vi "Monitor Torque 2.vi"(0 "reference in":refnum<class "SmartMotor.lvclass">, 3 "Monitoring Duration (ms)":u32, 4 "Torque Limit":i32, 5 "error in (no error)":errorcluster) -> (14 "reference out":refnum<class "SmartMotor.lvclass">, 18 "Limit Passed":bool, 19 "error out":errorcluster)   [LabVIEW 2017, in "SmartMotor.lvclass"]
uses:
  SmartMotor.lvclass
  <vilib>/Analysis/baseanly.llb/Mean (DBL).vi
  <vilib>/Analysis/NI_AALBase.lvlib
panel:
  out "Absolute Motor Torque":dbl(graph)
  out "Max Absolute Torque":dbl
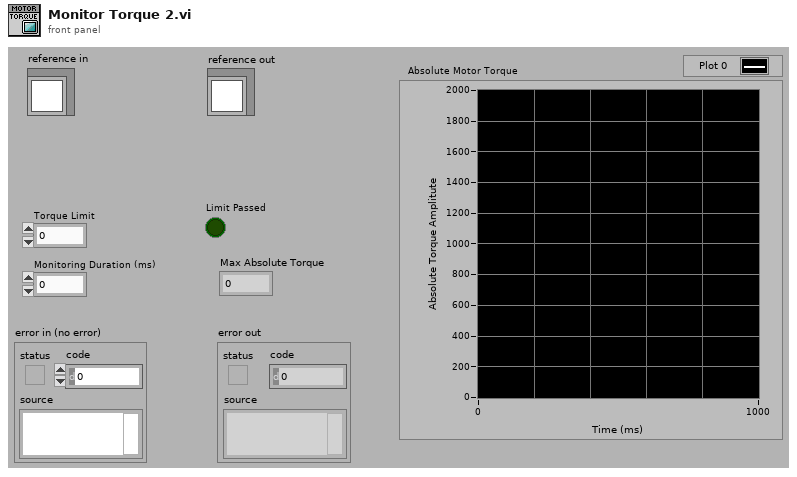
[diagram p1: front panel]
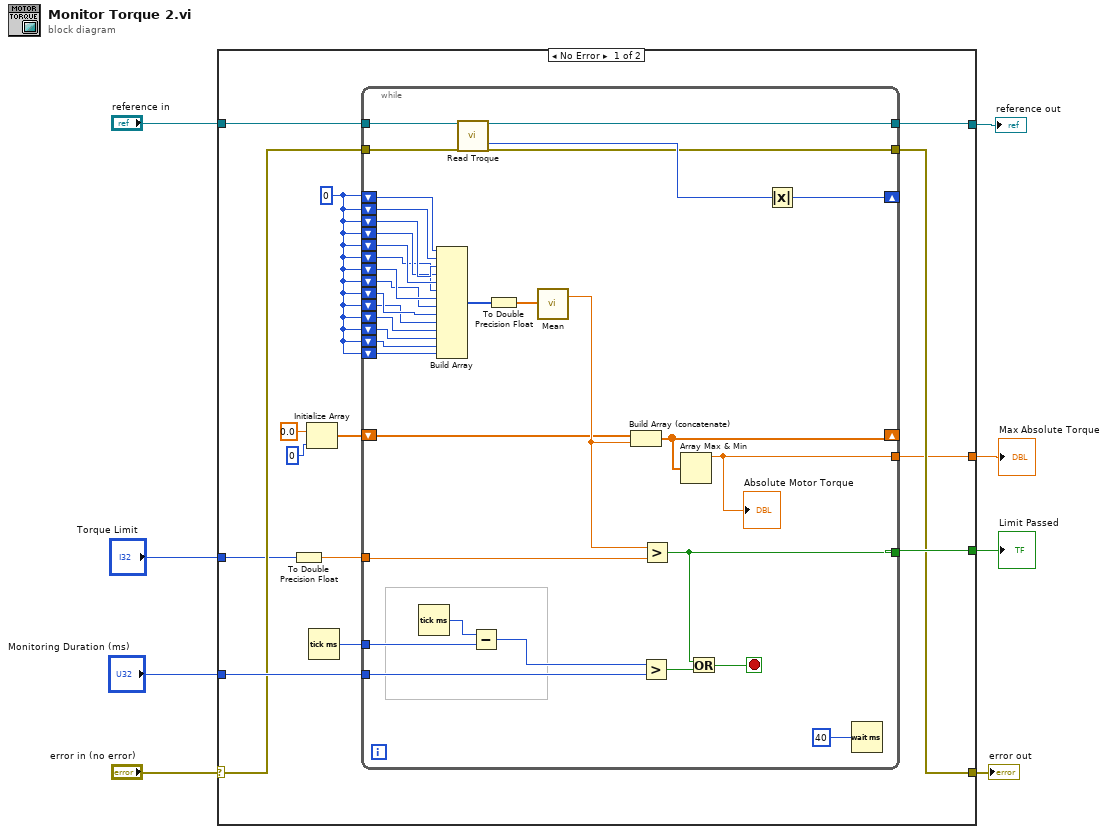
[diagram p0: block diagram]
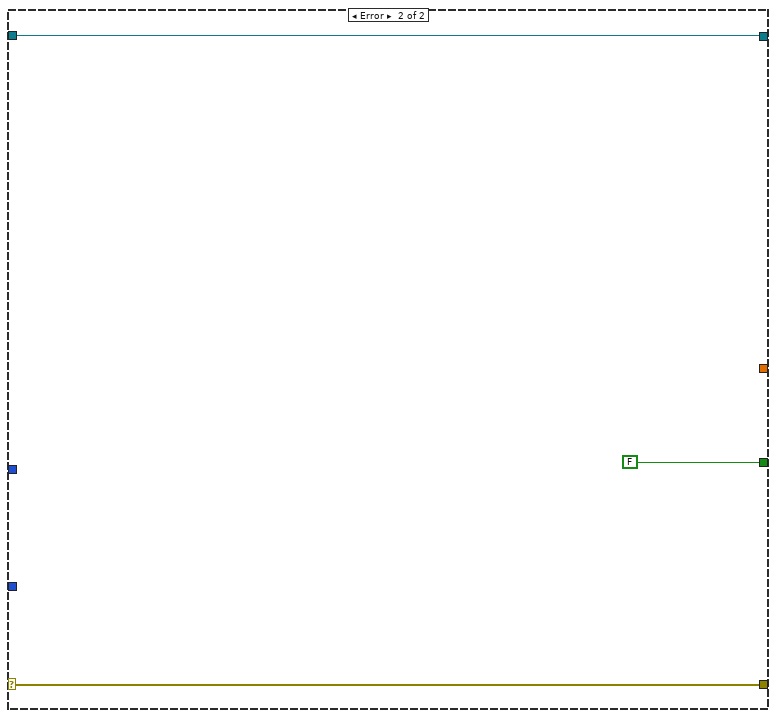
[diagram p2: hidden frame]
diagram:
  n1 = case shown="No Error" "error in (no error)" {
    selector: "error in (no error)" -> [w18 w60]
    tunnel: [w17 w60] -> w7
    tunnel: [w16 w59] -> w5
    tunnel: "reference in" -> [w22 w59]
    tunnel: "Monitoring Duration (ms)" -> [w20 _]
    tunnel: "Torque Limit" -> [w14 _]
    tunnel: [w19 FALSE] -> w2
    tunnel: [w9 _] -> w1
    frame No Error {
      w15 = 0
      n2 = To Double Precision Float(number=w14) -> (double precision float=w13:dbl)
      n3 = Initialize Array(0.0 ("element"), 0 ("dimension size")) -> (w12:dbl[])
      n4 = Tick Count (ms)() -> (millisecond timer value=w21:u32)
      n5 = while {
        tunnel: w22 -> [w57]
        tunnel: w21 -> [w56]
        tunnel: w20 -> [w53]
        tunnel: [w49] -> w19
        tunnel: w18 -> [w48]
        tunnel: [w47] -> w17
        tunnel: [w46] -> w16
        shift-right: [w29] -> _
        shift-left: w15 -> [w45]
        shift-left: w15 -> [w44]
        shift-left: w15 -> [w43]
        shift-left: w15 -> [w42]
        shift-left: w15 -> [w41]
        shift-left: w15 -> [w40]
        shift-left: w15 -> [w39]
        shift-left: w15 -> [w38]
        shift-left: w15 -> [w37]
        shift-left: w15 -> [w36]
        shift-left: w15 -> [w35]
        shift-left: w15 -> [w34]
        shift-left: w15 -> [w33]
        shift-left: w15 -> [w32]
        tunnel: w13 -> [w28]
        shift-right: [w25] -> _
        shift-left: w12 -> [w26]
        tunnel: [w24] -> w9
        stop <- w50 stop-if-true
        n6 = Tick Count (ms)() -> (millisecond timer value=w55:u32)
        n7 = Build Array(w45, w44, w43, w42, w41, w40, w39, w38, w37, w36, w35, w34, w33, w32) -> (w30:i32[])
        n8 = call-dynamic "Read Troque.vi"("reference in"=w57, "error in (no error)"=w48) -> ("reference out"=w46:refnum<class "SmartMotor.lvclass">, "Motor Torque"=w52:i32, "error out"=w47:errorcluster)  [unwired: 15 in]
        n9 = Subtract(x=w55, y=w56) -> (x-y=w54:u32)
        n10 = To Double Precision Float(number=w30) -> (double precision float=w31:dbl[])
        n11 = call-poly <vilib>:"Mean.vi"("X"=w31) -> ("mean"=w27:dbl)  [unwired: 1 out]
        n12 = Build Array (concatenate)(w26, w27) -> (w25:dbl[])
        n13 = Greater?(x=w54, y=w53) -> (0:w51:bool)
        n14 = Greater?(x=w27, y=w28) -> (0:w49:bool)
        n15 = Array Max & Min(array=w25) -> (max value=w24:dbl)  [unwired: 3 out]
        "Absolute Motor Torque" <- w24
        n16 = Or(x=w49, y=w51) -> (x .or. y?=w50:bool)
        n17 = Absolute Value(x=w52) -> (abs(x)=w29:i32)
        n18 = Wait (ms)(milliseconds to wait=u32 40) -> ()  [unwired: 1 out]
      }
    }
    frame Error {
    }
  }
  "error out" <- w7
  "reference out" <- w5
  "Limit Passed" <- w2
  "Max Absolute Torque" <- w1
